vi "AutofocusOptions.vi"() -> ()   [LabVIEW 2019]
uses:
  <vilib>/Utility/file.llb/Read Delimited Spreadsheet (DBL).vi
panel:
  out "N_iterations":dbl[](array[numeric])
  in  "InitialStepSize":dbl=0.1
  out "HighVSPosition":picture
  in  "Z OutputFile":path=path "C:/Users/TTUHEP/Documents/LabVIEW/GantryPrograms/Configs/temp.txt"
  in  "Plot Output File":string="C:\\Users\\TTUHEP\\Documents\\LabVIEW\\GantryPrograms\\LogFiles\\plot.png"
  out "spreadsheet string":string
  in  "Radius":dbl
  in  "Center Position":string
  out "Image":T1(plugin-control)
  in  "InitialPositions":path=path "C:/Users/TTUHEP/Documents/LabVIEW/GantryPrograms/Configs/BasePlateEdgesA1.txt"
  out "error out":errorcluster
  out "Best Z value":dbl
  in  "Filter Type":T2(ring)=enum."Sobel"
  in  "error in (no error)":errorcluster
  in  "SpeedZ (mm/s)":dbl=10.0
  in  "SpeedXY (mm/s)":dbl=100.0
  in  "Z":dbl=68.683
  in  "Y":dbl=948.353
  in  "X":dbl=295.755
  in  "ControlType":T3(ring)=enum."Text File" caption="Operation Mode"
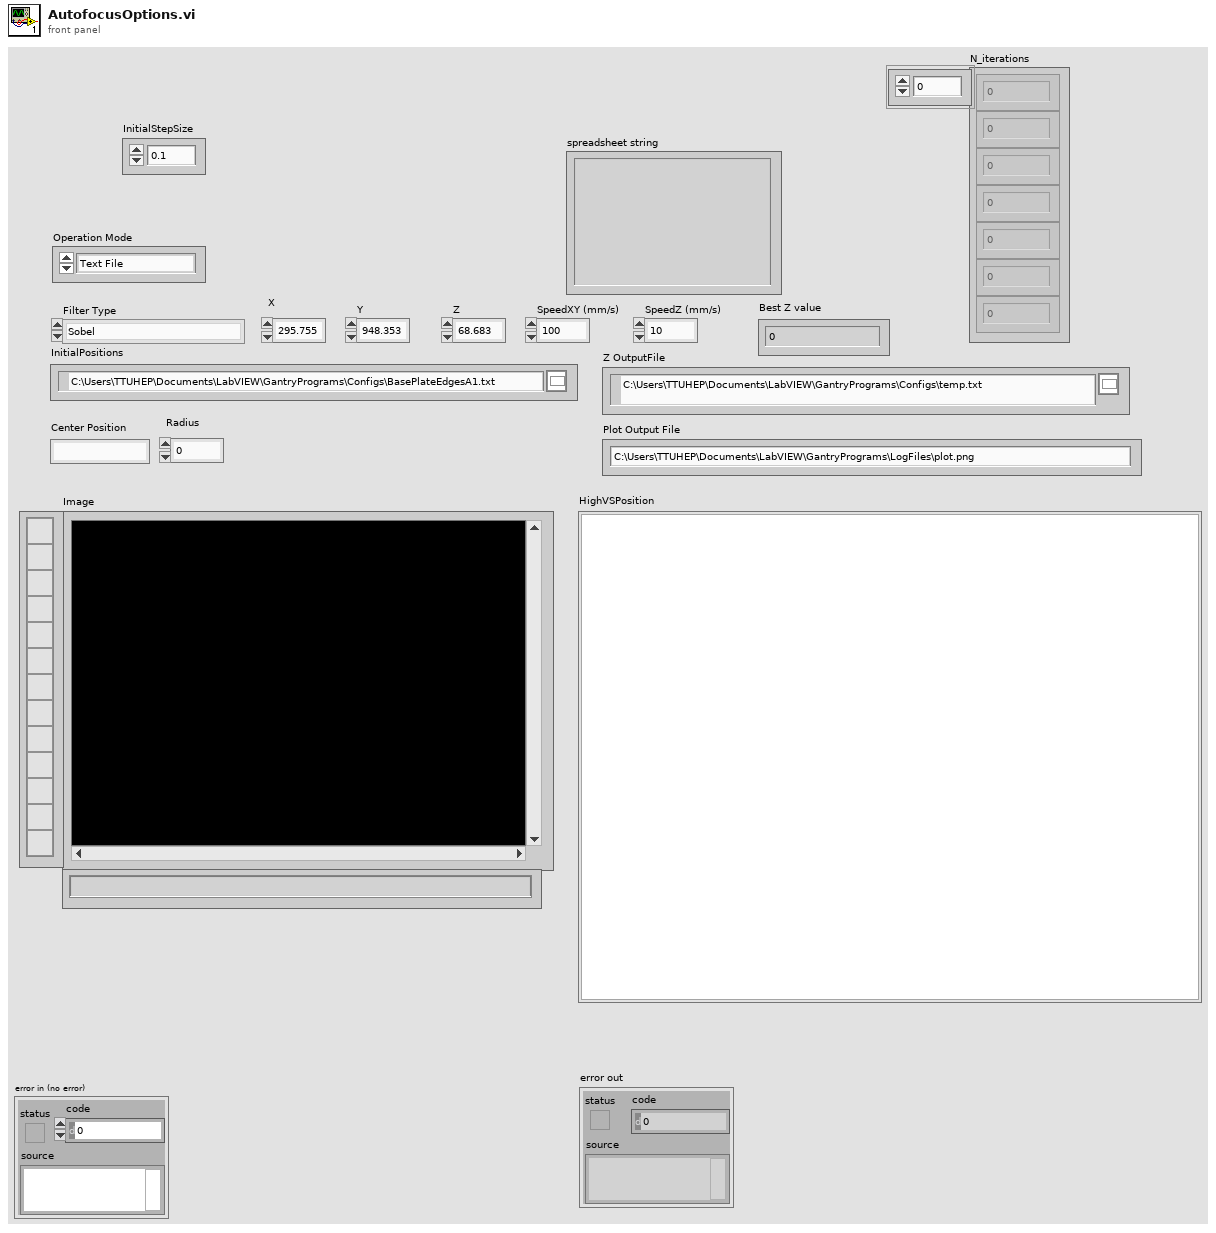
[diagram p1: front panel]
types:
  T1 = typedef "IMAQ Image.ctl" = refnum<image>
  T2 = enum16{"Convolution", "Differentiation", "Gradient", "Prewitt", "Roberts", "Sigma", "Sobel"}
  T3 = enum16{"Single Point Measurement", "Text File", "Measurements in a circle"}
  T4 = enum16{"open", "replace", "create", "open or create", "replace or create", "replace or create with confirmation"}
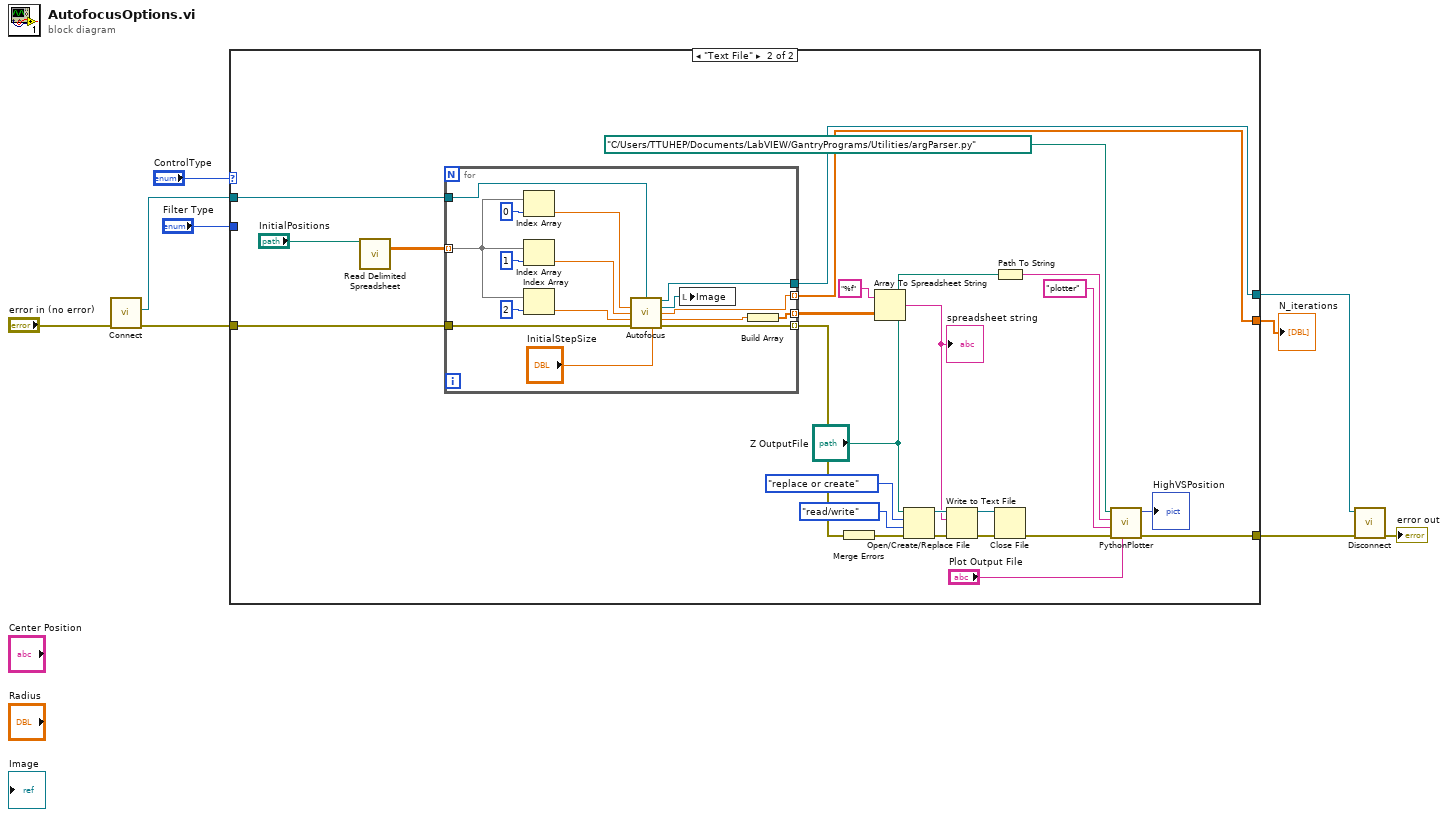
[diagram p0: block diagram]
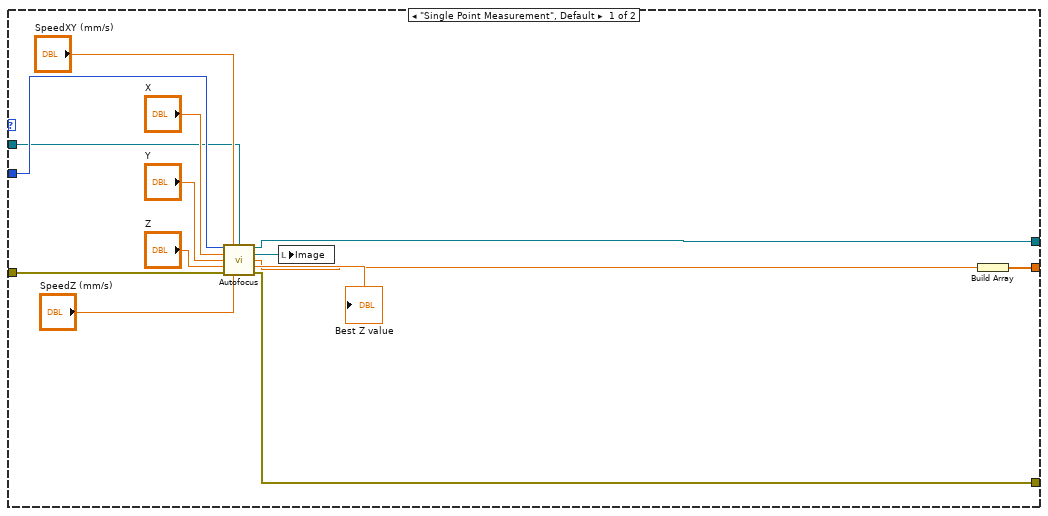
[diagram p2: hidden frame]
diagram:
  n1 = call "Connect.vi"("error in (no error)"="error in (no error)") -> ("error out"=w5:errorcluster, "controller"=w7:refnum<k24>)  [unwired: 9 in]
  n2 = case shown="\"Text File\"" "ControlType" {
    tunnel: w5 -> [w18 w46]
    tunnel: "Filter Type" -> [w17 _]
    tunnel: [w15 w26] -> w4
    tunnel: w7 -> [w14 w44]
    tunnel: [w13 w43] -> w2
    tunnel: [w10 w24] -> w1
    frame "Single Point Measurement", Default {
      n3 = call "Autofocus.vi"("Filter Type"=w17, "SpeedXY (mm/s)"="SpeedXY (mm/s)", "controller in"=w14, "X"="X", "Y"="Y", "Z"="Z", "error in (no error)"=w18, "SpeedZ (mm/s)"="SpeedZ (mm/s)") -> ("controller out"=w13:refnum<k24>, "Image"=w12:T1, "N_iterations"=w11:dbl, "BestZvalue"=→"Best Z value":dbl, "error out"=w15:errorcluster)  [unwired: 3 in]
      n4 = local write "Image"(w12) -> ()
      n5 = Build Array(w11) -> (w10:dbl[])
    }
    frame "Text File" {
      n6 = call-poly <vilib>:"Read Delimited Spreadsheet.vi"("file path (dialog if empty)"="InitialPositions") -> ("all rows"=w48:dbl[][])  [unwired: 9 in, 5 out]
      n7 = for {
        tunnel: w48 -> [w61] mode=indexing
        tunnel: w46 -> [w56]
        tunnel: [w55] -> w45 mode=indexing
        tunnel: [w54] -> w42 mode=indexing
        tunnel: w44 -> [w53]
        tunnel: [w52] -> w43
        tunnel: [w49] -> w24 mode=indexing
        n8 = Index Array(array=w61, index=0) -> (element=w60:dbl)
        n9 = Index Array(array=w61, index=1) -> (element=w59:dbl)
        n10 = Index Array(array=w61, index=2) -> (element=w58:dbl)
        n11 = call "Autofocus.vi"("controller in"=w53, "X"=w60, "Y"=w59, "Z"=w58, "error in (no error)"=w56, "InitialStepSize"="InitialStepSize") -> ("controller out"=w52:refnum<k24>, "Image"=w51:T1, "N_iterations"=w49:dbl, "BestZvalue"=w57:dbl, "error out"=w55:errorcluster)  [unwired: 5 in]
        n12 = local write "Image"(w51) -> ()
        n13 = Build Array(w57) -> (w54:dbl[])
      }
      n14 = Merge Errors(w45) -> (w28:errorcluster)
      n15 = Array To Spreadsheet String(array=w42, 3:"%f" ("format string")) -> (spreadsheet string=w31:string)  [unwired: 1 in]
      "spreadsheet string" <- w31
      n16 = Open/Create/Replace File(file path (use dialog)="Z OutputFile", error in=w28, operation (0:open)=T4."replace or create", access (0:read/write)=enum16{"read/write", "read-only", "write-only"}."read/write") -> (refnum out=w34:refnum<file>, error out=w35:errorcluster)  [unwired: 2 in, 1 out]
      n17 = Write to Text File(file (use dialog)=w34, text=w31, error in=w35) -> (refnum out=w37:refnum<file>, error out=w36:errorcluster)  [unwired: 1 in, 1 out]
      n18 = Path To String(path="Z OutputFile") -> (string=w29:string)
      n19 = Close File(refnum=w37, error in=w36) -> (error out=w27:errorcluster)  [unwired: 1 out]
      n20 = call "PythonPlotter.vi"("Output File"="Plot Output File", "error in (no error)"=w27, "Function Name"="plotter", "Input File"=w29, "Python Path"=path "C:/Users/TTUHEP/Documents/LabVIEW/GantryPrograms/Utilities/argParser.py") -> ("error out"=w26:errorcluster, "HighVSPosition"=→"HighVSPosition":picture)  [unwired: 4 in]
    }
  }
  "N_iterations" <- w1
  n21 = call "Disconnect.vi"("error in (no error)"=w4, "controller"=w2) -> ("error out"=→"error out":errorcluster)  [unwired: 9 in]
